vi "3458A Close Virtual Channels.vi"(8 "error in":errorcluster, 10 "Reset to preset mode (True)":bool=TRUE, 11 "session in":T1 {"channels"."Range [Vpk]" min=0.0}) -> (0 "error out":errorcluster, 3 "session out":T1 {"channels"."Range [Vpk]" min=0.0})   [LabVIEW 2018, in "3458A Virtual Digitizer.lvlib"]
doc: "Call this to close all instruments related to the opened session. It automatically does cleanup of digitizing processes, i.e. stops them, destroys data queues and notifiers."
uses:
  3458A Virtual Digitizer.lvlib
  3458A Digitizer Session.ctl
  3458A Virtual Channel Config.ctl
  Counter/Counter Session.ctl
  Counter/Counter Type.ctl
  AWG/AWG Session.ctl
  AWG/AWG Type.ctl
  3458A Sync Mode.ctl
  3458A Idn Mode.ctl
  3458A Digitizing Low Levels/Configure/Sampling Mode.ctl
  3458A Digitizing Process Options.ctl
  3458A Data Packet.ctl
  3458A Aux Record Data.ctl
  3458A Digitizing Low Levels/Configure/Level Setup.ctl
  3458A Digitizing Low Levels/Configure/First Sample Trigger.ctl
  3458A Aperture Selection Mode.ctl
  3458A Digitizing Low Levels/3458A Digitizing Low Levels.lvlib
  AWG/AWG.lvlib
  Counter/Counter.lvlib
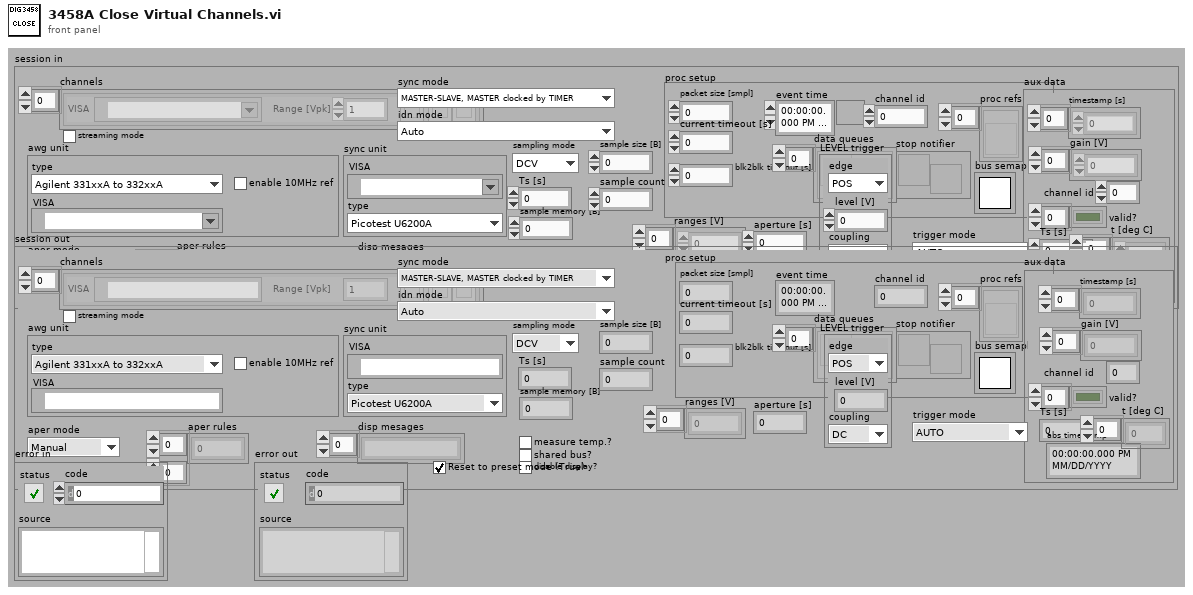
[diagram p1: front panel]
types:
  T1 = typedef "3458A Virtual Digitizer.lvlib/3458A Digitizer Session.ctl" = cluster{"channels":T2[], "sync unit":T3, "awg unit":T5, "sync mode":T7, "streaming mode":bool, "idn mode":T8, "sampling mode":T9, "Ts [s]":dbl, "sample memory [B]":i32, "proc setup":T10, "sample size [B]":i32, "sample count":i32, "aux data":T12, "ranges [V]":dbl[], "aperture [s]":dbl, "LEVEL trigger":T13, "trigger mode":T14, "measure temp.?":bool, "disp mesages":string[], "shared bus?":bool, "disable display?":bool, "aper mode":T15, "aper rules":dbl[][]}
  T2 = typedef "3458A Virtual Digitizer.lvlib/3458A Virtual Channel Config.ctl" = cluster{"VISA":refnum<visa-resource-name>, "Range [Vpk]":dbl, "btn clr":bool, "btn up":bool, "btn down":bool}
  T3 = typedef "Counter.lvlib/Counter Session.ctl" = cluster{"VISA":refnum<visa-resource-name>, "type":T4}
  T4 = typedef "Counter.lvlib/Counter Type.ctl" = enum16{"Picotest U6200A", "dummy"}
  T5 = typedef "AWG.lvlib/AWG Session.ctl" = cluster{"type":T6, "VISA":refnum<visa-resource-name>, "enable 10MHz ref":bool}
  T6 = typedef "AWG.lvlib/AWG Type.ctl" = enum16{"Agilent 331xxA to 332xxA", "Agilent 335xxA to 336xxA", "Tektronix AFG3101C", "dummy"}
  T7 = typedef "3458A Virtual Digitizer.lvlib/3458A Sync Mode.ctl" = enum16{"MASTER-SLAVE, MASTER clocked by TIMER", "MASTER-SLAVE, MASTER clocked by AWG", "ALL clocked by AWG", "MASTER-SLAVE, ALL clocked by TIMER", "ALL clocked by AWG with DFLL"}
  T8 = typedef "3458A Virtual Digitizer.lvlib/3458A Idn Mode.ctl" = enum16{"Auto", "Sequential (chn A, chn B, ...)", "From calibration string"}
  T9 = typedef "3458A Virtual Digitizer.lvlib/3458A Digitizing Low Levels.lvlib/Sampling Mode.ctl" = enum16{"DCV", "DSDC", "DSAC"}
  T10 = typedef "3458A Virtual Digitizer.lvlib/3458A Digitizing Process Options.ctl" = cluster{"channel id":i32, "packet size [smpl]":i32, "current timeout [s]":dbl, "blk2blk timeout [s]":dbl, "event time":timestamp, "stop notifier":refnum<notifier>, "data queues":refnum<queue>[], "proc refs":refnum<vi>[], "bus semaphore":T11}
  T11 = typedef "Semaphore RefNum" = refnum<k1>
  T12 = typedef "3458A Virtual Digitizer.lvlib/3458A Aux Record Data.ctl" = cluster{"channel id":i32, "valid?":bool[], "gain [V]":dbl[], "timestamp [s]":dbl[], "Ts [s]":dbl, "abs timestamp":timestamp, "t [deg C]":dbl[]}
  T13 = typedef "3458A Virtual Digitizer.lvlib/3458A Digitizing Low Levels.lvlib/Level Setup.ctl" = cluster{"edge":enum16{"POS", "NEG"}, "level [V]":dbl, "coupling":enum16{"DC", "AC"}}
  T14 = typedef "3458A Virtual Digitizer.lvlib/3458A Digitizing Low Levels.lvlib/First Sample Trigger.ctl" = enum16{"AUTO", "EXT", "SYN", "SGL", "HOLD", "LEVEL"}
  T15 = typedef "3458A Virtual Digitizer.lvlib/3458A Aperture Selection Mode.ctl" = enum16{"Manual", "Maximum", "Table"}
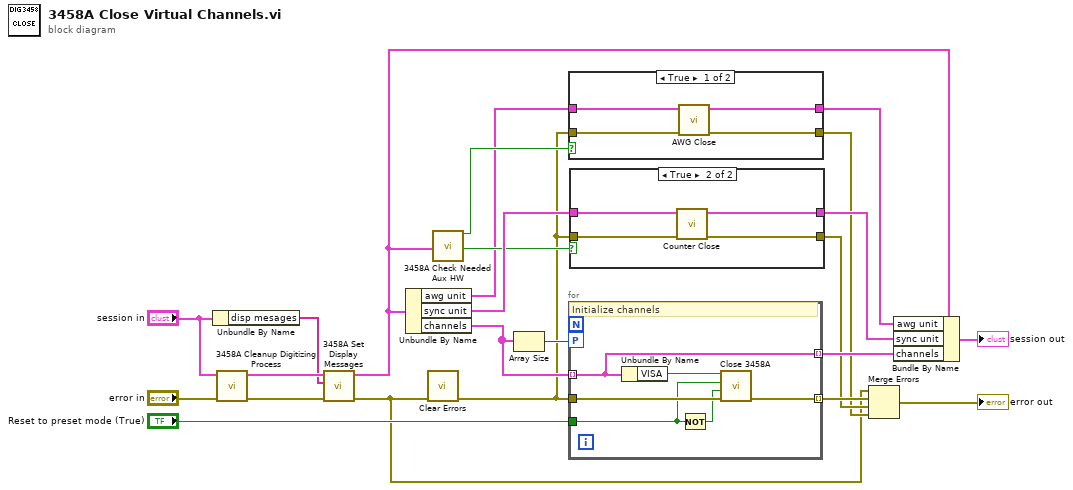
[diagram p0: block diagram]
diagram:
  n1 = Unbundle By Name("session in") -> ("disp mesages"=w1:string[])
  n2 = call "3458A Cleanup Digitizing Process.vi"("error in"="error in", "session in"="session in") -> ("error out"=w6:errorcluster, "session out"=w4:T1)  [unwired: 8 in]
  n3 = call "3458A Set Display Messages.vi"("error in (no error)"=w6, "display strings"=w1, "digitizer session in"=w4) -> ("error out"=w5:errorcluster, "digitizer session out"=w3:T1)  [unwired: 7 in]
  n4 = Unbundle By Name(w3) -> ("awg unit"=w8:T5, "sync unit"=w20:T3, "channels"=w23:T2[])
  n5 = call <vilib>:"Clear Errors.vi"("error in (no error)"=w5) -> ("error out"=w7:errorcluster)  [unwired: 5 in, 1 out]
  n6 = call "3458A Check Needed Aux HW.vi"("digitizer session"=w3) -> ("uses AWG clocking?"=w11:bool, "uses counter?"=w12:bool)  [unwired: 13 in, 4 out]
  n7 = Array Size(array=w23) -> (size(s)=w22:i32)
  n8 = case shown="True" w11 {
    tunnel: w7 -> [w27 w29]
    tunnel: [w24 w29] -> w10
    tunnel: w8 -> [w26 w28]
    tunnel: [w25 w28] -> w9
    frame True {
      # "Initialize AWG"
      n9 = call "AWG Close.vi"("error in (no error)"=w27, "awg session in"=w26) -> ("error out"=w24:errorcluster, "awg session out"=w25:T5)  [unwired: 8 in]
    }
    frame False {
    }
  }
  n10 = for {
    tunnel: w7 -> [w35]
    tunnel: w23 -> [w32] mode=indexing
    workers-P: w22 -> [_]
    tunnel: [w34] -> w21 mode=indexing
    tunnel: [w32] -> w18 mode=indexing
    tunnel: "Reset to preset mode (True)" -> [w30]
    # "Initialize channels"
    n11 = Unbundle By Name(w32) -> ("VISA"=w33:refnum<visa-resource-name>)
    n12 = Not(x=w30) -> (.not. x?=w31:bool)
    n13 = call "Close 3458A.vi"("error in (no error)"=w35, "keep display in whatever mode? (False)"=w31, "Reset to preset mode (True)"=w30, "VISA resource name"=w33) -> ("error out"=w34:errorcluster)  [unwired: 7 in]
  }
  n14 = case shown="True" w12 {
    tunnel: w7 -> [w36 w41]
    tunnel: w20 -> [w37 w40]
    tunnel: [w36 w38] -> w17
    tunnel: [w37 w39] -> w19
    frame False {
      # "Initialize AWG"
    }
    frame True {
      # "Initialize counter"
      n15 = call "Counter Close.vi"("error in"=w41, "couner session in"=w40) -> ("error out"=w38:errorcluster, "counter session out"=w39:T3)  [unwired: 8 in]
    }
  }
  n16 = Merge Errors(w5, w21, w17, w10) -> (→"error out":errorcluster)
  n17 = Bundle By Name(cluster=w3, "awg unit"=w9, "sync unit"=w19, "channels"=w18) -> (→"session out":T1)
